vi "EV3Tests.vi"() -> ()   [LabVIEW 2019]
uses:
  <userlib>/MicroPython/VIs/uPythonX/uPythonX.xctl
panel:
  in  "PYBD 2":T1(xcontrol)={"VISA Refnum in"="HighPeaksPYBD - ASRL114::INSTR", "Python Code"="import gc,utime\nimport pyb, micropython\nimport LPF2\n\nmicropython.alloc_emergency_exception_buf(200)\n\nmodes = [\nLPF2.mode('US-DIST-CM',type = LPF2.DATA16),\n]\n\nred_led=pyb.LED(1)\ngreen_led = pyb.LED(2)\nred_led.on()\n\nlpf2 = LPF2.EV3_LPF2(1, 'Y1', 'Y2', modes, 30, timer = 4, freq = 5)    # PyBoard\n\nlpf2.initialize()\n\nvalue = 0\n\n# Loop\nwhile True:\n     if not lpf2.connected:\n          lpf2.sendTimer.callback(None)\n          red_led.on()\n          utime.sleep_ms(200)\n          lpf2.initialize()\n     else:\n          red_led.off()\n          \n          if lpf2.current_mode == 0:\n               lpf2.load_payload('Int16',9)\n          else:\n               lpf2.load_payload('Int16',5)\n\n          utime.sleep_ms(90)\n          \n"}
  in  "Beep + LPF2":T2(xcontrol)={"Port"="130.64.157.92", "All Code"="#!/usr/bin/env pybricks-micropython\n\nfrom pybricks import ev3brick as brick\nfrom pybricks.ev3devices import (Motor, TouchSensor, ColorSensor,\n                                 InfraredSensor, UltrasonicSensor, GyroSensor)\nfrom pybricks.parameters import (Port, Stop, Direction, Button, Color,\n                                 SoundFile, ImageFile, Align)\nfrom pybricks.tools import print, wait, StopWatch\nfrom pybricks.robotics import DriveBase\n\n# Write your program here\nbrick.sound.beep()\n\ndist=UltrasonicSensor(Port.S4)\nprint(dist.distance())"}
  in  "Sound and Light":T3(xcontrol)={"VISA Refnum in"="169.254.29.229", "All Code"="#!/usr/bin/env pybricks-micropython\n\nfrom pybricks import ev3brick as brick\nfrom pybricks.parameters import Button, Color,ImageFile\nfrom pybricks.tools import print, wait\n\n# Write your program here\n# A high pitch (1500 Hz) for one second (1000 ms) at 50% volume\nbrick.sound.beep(500, 1000, 20)\n\nbrick.light(Color.RED)\nLight = [Color.BLACK, Color.GREEN, Color.YELLOW, Color.RED, Color.ORANGE]\n\nfor color in Light:\n    print(color)\n    try:\n        brick.light(color)\n    except:\n        print('bad')\n    wait(500)\n\nbrick.display.clear()\nbrick.display.text(brick.battery.voltage(), (0, 50))\nwhile not Button.CENTER in brick.buttons():\n    wait(100)\nbrick.display.image(ImageFile.UP)\nwhile not Button.CENTER in brick.buttons():\n    wait(100)\n\nwhile True:\n    # Do something if the left button is pressed\n    if Button.LEFT in brick.buttons():\n        print(\"The left button is pressed.\")\n        break\n    wait(100)"}
  # "Errors:\n1. IP address does nto get passed back\n2. sometimes it does not send lines out - lines get lost somewhere..."
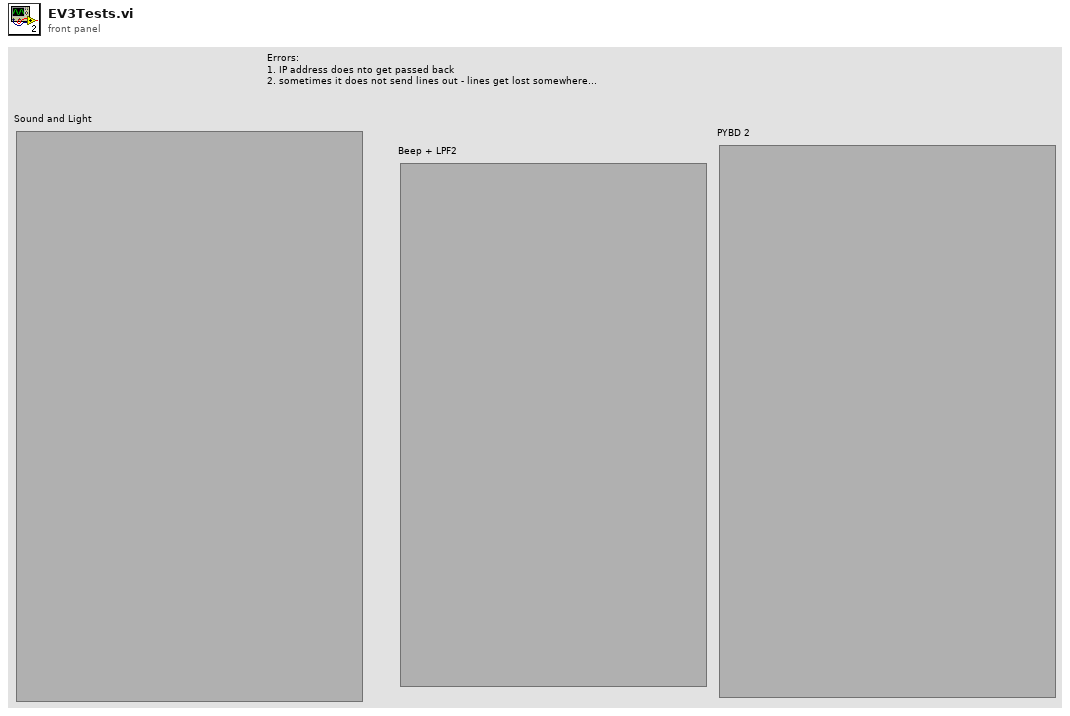
[diagram p1: front panel]
types:
  T1 = cluster{"VISA Refnum in":refnum<visa-resource-name>, "Python Code":string}
  T2 = cluster{"Port":refnum<visa-resource-name>, "All Code":string}
  T3 = cluster{"VISA Refnum in":refnum<visa-resource-name>, "All Code":string}
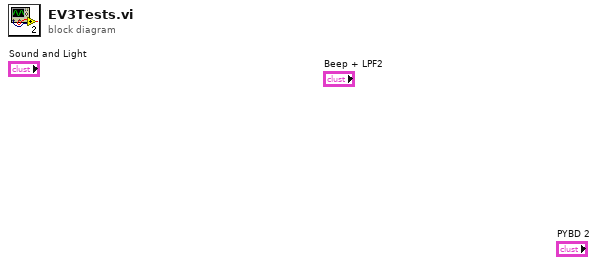
[diagram p0: block diagram]
diagram:
